vi "Test_WriteAandBandC_ListAll_ReturnAandBandC.vi"(8 "error in (no error)":errorcluster, 11 "TestCase in":refnum<class "TestComposedLookupTable.lvclass">) -> (0 "error out":errorcluster, 3 "TestCase out":refnum<class "TestComposedLookupTable.lvclass">)   [LabVIEW 2017, in "TestComposedLookupTable.lvclass"]
uses:
  TestComposedLookupTable.lvclass
  Source/LookupTable/LookupTable.lvclass/LookupTable.ctl
  814f90a6-7759-4b35-9e29-8985ceb8ac39.vi
  Source/LookupTable/Read Table Reference.vi
  814f90a6-7759-4b35-9e29-8985ceb8ac39.vi/b1c1744f-f4ec-4f7c-9c9d-24e90e18623c.vi
  Source/LookupTable/LookupTable.lvclass
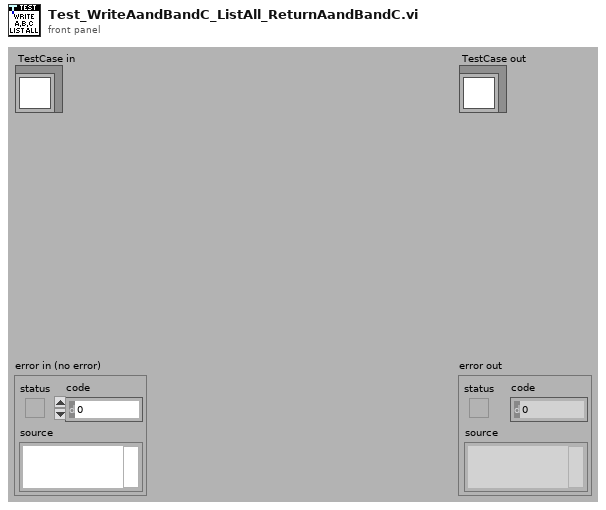
[diagram p1: front panel]
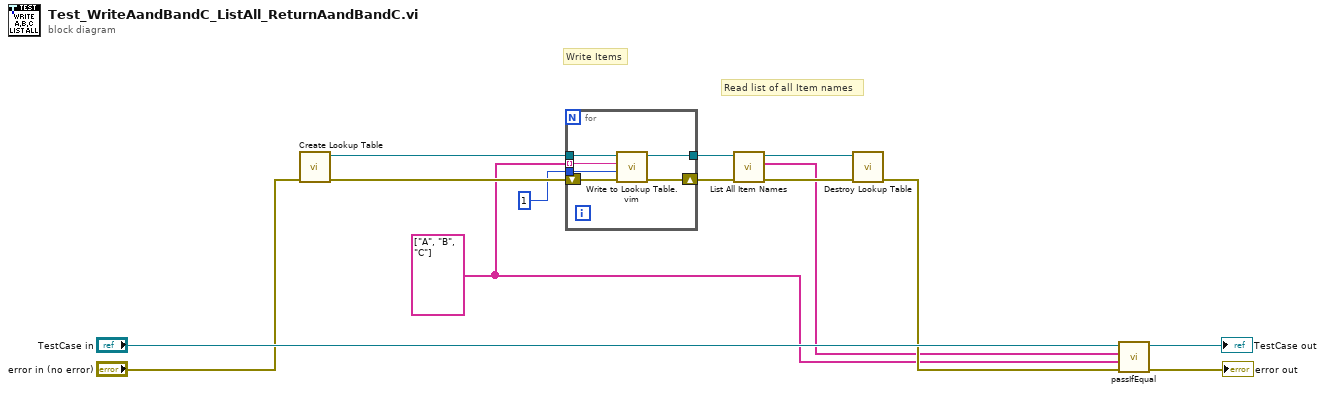
[diagram p0: block diagram]
diagram:
  w2 = string[] ["A", "B", "C"] ("Item Name")
  # "Read list of all Item names"
  # "Write Items"
  n1 = call "Create Lookup Table.vi"("error in (no error)"="error in (no error)") -> ("error out"=w14:errorcluster, "LookupTable Reference"=w10:refnum<data-value>)  [unwired: 9 in]
  n2 = for {
    tunnel: w2 -> [w19] mode=indexing
    tunnel: w10 -> [w18]
    tunnel: 1 -> [w17]
    tunnel: [w16] -> w4
    shift-right: [w15] -> w6
    shift-left: w14 -> [w20]
    n3 = call "Write to Lookup Table.vim"("error in (no error)"=w20, "Item"=w17, "Item Name"=w19, "LookupTable Reference"=w18) -> ("error out"=w15:errorcluster, "LookupTable Reference Out"=w16:refnum<data-value>)  [unwired: 5 in, 1 out]
  }
  n4 = call "List All Item Names.vi"("error in (no error)"=w6, "LookupTable Reference"=w4) -> ("error out"=w5:errorcluster, "All Items"=w1:string[], "LookupTable Reference Out"=w3:refnum<data-value>)  [unwired: 6 in, 1 out]
  n5 = call "Destroy Lookup Table.vi"("error in (no error)"=w5, "LookupTable Reference"=w3) -> ("error out"=w8:errorcluster)  [unwired: 9 in]
  n6 = call-dynamic "passIfEqual.vi"("error in (no error)"=w8, "y"=w2, "x"=w1, "TestCase in"="TestCase in") -> ("error out"=→"error out":errorcluster, "TestCase out"=→"TestCase out":refnum<class "TestComposedLookupTable.lvclass">)  [unwired: 6 in]
